vi "TS530A_give_SetPoint_light.vi"(0 "Set Point":i32=1 min=1 max=40000 step=1, 1 "dup VISA session":refnum<visa-resource-name>, 2 "ObAllein":bool, 3 "PROPORTIONAL GAIN":i8=-1 min=-1 max=15, 4 "INTEGRATOR TC":i8=-1 min=-1 max=11, 6 "DERIVATOR TC":i8=-1 min=-1 max=7, 9 "HEATER POWER RANGE":i8=-1 min=-1 max=7, 10 "POWER BIAS":i8=-1 min=-1 max=5) -> (7 "set point":dbl, 8 "dup VISA session 2":refnum<visa-resource-name>)   [LabVIEW 2010]
uses:
  Programme/National Instruments/LabVIEW 8.5/instr.lib/Mischerinstr.lib/AVS-Brücke/LV Drivers for AVS/AVS47IB.LLB/AVS47IB Wait for OPC/MAV/TMO.vi
panel:
  in  "error out":errorcluster
  in  "Case Constant\n(See Context Help)":bool
  out "TS 530A":bool
  in  "controll from \nSensor-Config.vi ?":bool
  in  "Sensor":u16(ring) items=["R4", "R6 RuOx", "nix", "nix", "nix", "nix"]
  out "Boolean":bool=TRUE
  out "Delta t (sec)":u32 format="%.2f"
  out "millisecond \ntimer value":u32
  out "Iter.Nr":i32
  in  "stop":bool
  in  "GPIB addr":u8=20 min=1 max=32 step=1
  # "(1 ~ 19999)"
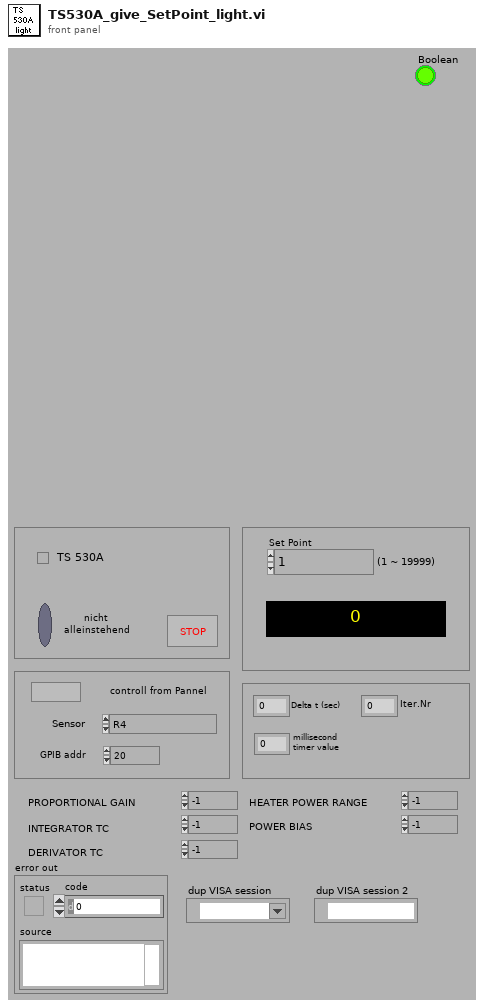
[diagram p1: front panel]
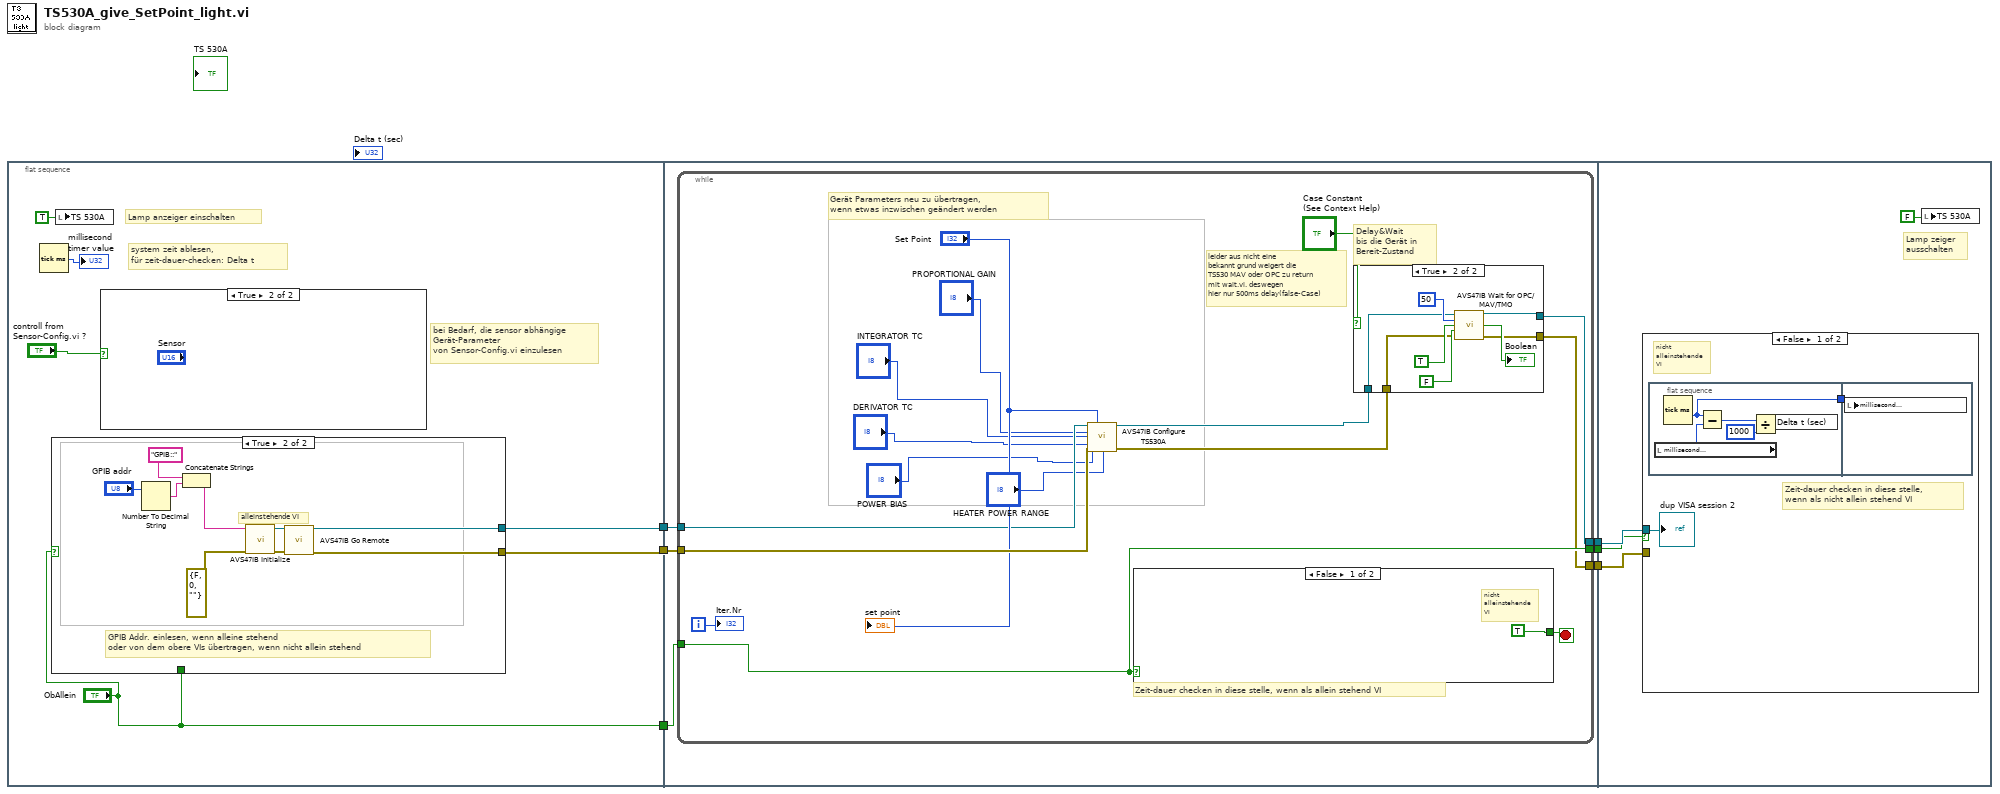
[diagram p0: block diagram]
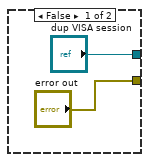
[diagram p2: hidden frame]
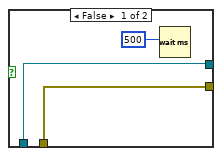
[diagram p4: hidden frame]
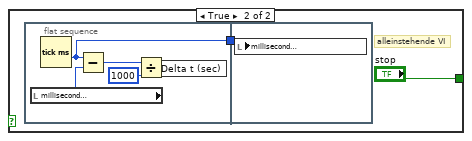
[diagram p5: hidden frame]
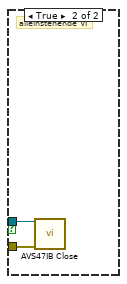
[diagram p6: hidden frame]
diagram:
  n1 = flat-sequence {
    tunnel: [w10] -> w6
    tunnel: ["ObAllein"] -> w3
    tunnel: [w11] -> w1
    tunnel: w6 -> [w29]
    tunnel: [w28] -> w5
    tunnel: [w27] -> w4
    tunnel: w3 -> [w26]
    tunnel: [w25] -> w2
    tunnel: w1 -> [w24]
    tunnel: w5 -> [w68]
    tunnel: w4 -> [w67]
    tunnel: w2 -> [w66]
    frame #0 {
      # "bei Bedarf, die sensor abhängige\nGerät-Parameter\nvon Sensor-Config.vi einzulesen"
      # "system zeit ablesen, \nfür zeit-dauer-checken: Delta t"
      # "Lamp anzeiger einschalten"
      n2 = Tick Count (ms)() -> (millisecond timer value=→"millisecond \ntimer value":u32)
      n3 = case shown="True" "ObAllein" {
        tunnel: ["dup VISA session" w22] -> w11
        tunnel: ["error out" w21] -> w10
        tunnel: "ObAllein" -> [_ _]
        frame False {
        }
        frame True {
          # "alleinstehende VI"
          # "GPIB Addr. einlesen, wenn alleine stehend\noder von dem obere VIs übertragen, wenn nicht allein stehend"
          n4 = Number To Decimal String(number="GPIB addr") -> (decimal integer string=w16:string)  [unwired: 1 in]
          n5 = Concatenate Strings("GPIB::", w16) -> (w18:string)
          n6 = call "AVS47IB Initialize.vi"("Instr. Descriptor (GPIB::)"=w18, "error in (no error)"=errorcluster {"status"=FALSE, "code"=0, "source"=""}) -> ("VISA session"=w19:refnum<visa-resource-name>, "error out"=w20:errorcluster)  [unwired: 12 in]
          n7 = call "AVS47IB Go Remote.vi"("VISA session"=w19, "error in (no error)"=w20) -> ("dup VISA session"=w22:refnum<visa-resource-name>, "error out"=w21:errorcluster)  [unwired: 12 in]
        }
      }
      n8 = local write "TS 530A"(TRUE) -> ()
      n9 = case shown="True" "controll from \nSensor-Config.vi ?" {
        frame False {
        }
        frame True {
        }
      }
    }
    frame #1 {
      n10 = while {
        tunnel: w29 -> [w44]
        tunnel: [w38] -> w28
        tunnel: [w36] -> w27
        tunnel: w26 -> [w42]
        tunnel: [w42] -> w25
        tunnel: w24 -> [w40]
        i -> [w43]
        stop <- w45 stop-if-true
        # "leider aus nicht eine\nbekannt grund weigert die  \nTS530 MAV oder OPC zu return \nmit wait.vi. deswegen\nhier nur 500ms delay(false-Case)"
        # "Delay&Wait\nbis die Gerät in \nBereit-Zustand"
        # "Gerät Parameters neu zu übertragen,\nwenn etwas inzwischen geändert werden"
        # "Zeit-dauer checken in diese stelle, wenn als allein stehend VI"
        n11 = call "AVS47IB Configure TS530A.vi"("VISA session"=w40, "SET POINT (-1:no change)"="Set Point", "PROPORTIONAL GAIN (-1:no change)"="PROPORTIONAL GAIN", "INTEGRATOR TC  (-1:no change)"="INTEGRATOR TC", "DERIVATOR TC (-1:no change)"="DERIVATOR TC", "error in (no error)"=w44, "POWER BIAS  (-1:no change)"="POWER BIAS", "HEATER POWER RANGE  (-1:no change)"="HEATER POWER RANGE") -> ("dup VISA session"=w39:refnum<visa-resource-name>, "error out"=w37:errorcluster)  [unwired: 6 in]
        n12 = case shown="False" w42 {
          tunnel: [TRUE "stop"] -> w45
          frame False {
            # "nicht \nalleinstehende\nVI"
          }
          frame True {
            # "alleinstehende VI"
            n13 = flat-sequence {
              tunnel: [w63] -> w58
              tunnel: w58 -> [w65]
              frame #0 {
                n14 = local read "millisecond \ntimer value"() -> (w64:u32)
                n15 = Tick Count (ms)() -> (millisecond timer value=w63:u32)
                n16 = Subtract(x=w63, y=w64) -> (x-y=w62:u32)
                n17 = Divide(x=w62, y=1000) -> (x/y=w60:dbl)
                n18 = local write "Delta t (sec)"(w60) -> ()
              }
              frame #1 {
                n19 = local write "millisecond \ntimer value"(w65) -> ()
              }
            }
          }
        }
        n20 = case shown="True" "Case Constant\n(See Context Help)" {
          tunnel: w39 -> [w48 w52]
          tunnel: [w48 w51] -> w38
          tunnel: w37 -> [w47 w50]
          tunnel: [w47 w49] -> w36
          frame False {
            n21 = Wait (ms)(milliseconds to wait=500) -> ()  [unwired: 1 out]
          }
          frame True {
            n22 = call "AVS47IB Wait for OPC/MAV/TMO.vi"("VISA session"=w52, "Timeout (2 sec)"=50, "MAV (on)"=TRUE, "OPC (off)"=FALSE, "error in (no error)"=w50) -> ("dup VISA session"=w51:refnum<visa-resource-name>, "Timeout"=→"Boolean":bool, "error out"=w49:errorcluster)  [unwired: 8 in]
          }
        }
        "set point" <- "Set Point"
        "Iter.Nr" <- w43
      }
    }
    frame #2 {
      # "Lamp zeiger\nausschalten"
      n23 = case shown="False" w66 {
        tunnel: w68 -> [w70 w79]
        tunnel: w67 -> [_ w78]
        frame False {
          # "Zeit-dauer checken in diese stelle, \nwenn als nicht allein stehend VI"
          # "nicht \nalleinstehende\nVI"
          n24 = flat-sequence {
            tunnel: [w75] -> w71
            tunnel: w71 -> [w77]
            frame #0 {
              n25 = local read "millisecond \ntimer value"() -> (w76:u32)
              n26 = Tick Count (ms)() -> (millisecond timer value=w75:u32)
              n27 = Subtract(x=w75, y=w76) -> (x-y=w74:u32)
              n28 = Divide(x=w74, y=1000) -> (x/y=w72:dbl)
              n29 = local write "Delta t (sec)"(w72) -> ()
            }
            frame #1 {
              n30 = local write "millisecond \ntimer value"(w77) -> ()
            }
          }
          "dup VISA session 2" <- w70
        }
        frame True {
          # "alleinstehende VI"
          n31 = call "AVS47IB Close.vi"("VISA session"=w79, "error in (no error)"=w78) -> ()  [unwired: 13 in, 1 out]
        }
      }
      n32 = local write "TS 530A"(FALSE) -> ()
    }
  }
